vi "Set STG wrapper.vi"(7 "bAckEna":i32, 8 "error in (no error)":errorcluster caption="错误输入（无错误）", 9 "STG_INFO_OBJ In":T1={"uiSenNum"=1, "uiS1TrigerTime"=0, "uiS2TrigerTime"=0, "uiS3TrigerTime"=0} {"uiSenNum" items=["S1"=1, "S2"=2, "S3"=3]}, 10 "dwCanNodeId":u32, 11 "dwDevIndex":u32) -> (0 "error out":errorcluster caption="错误输出", 1 "STG_INFO_OBJ Out":T1={"uiSenNum"=1, "uiS1TrigerTime"=0, "uiS2TrigerTime"=0, "uiS3TrigerTime"=0} {"uiSenNum" items=["S1"=1, "S2"=2, "S3"=3]}, 3 "function return":u32)   [LabVIEW 2016, in "UISimCanFunc_wrapper.lvlib"]
doc: "_declspec (dllexport) DWORD SetSTG_wrapper(DWORD dwDevIndex, DWORD dwCanNodeId,\n P_STG_INFO_OBJ pStgInfoIn, BOOL bAckEna, P_STG_INFO_OBJ pStgInfoOut);"
uses:
  <userlib>/UISimCanFunc_wrapper/UISimCanFunc_wrapper.lvlib
  <userlib>/UISimCanFunc_wrapper/ctl/STG_INFO_OBJ.ctl
  <userlib>/UISimCanFunc_wrapper/UISimCanFunc_wrapper.dll
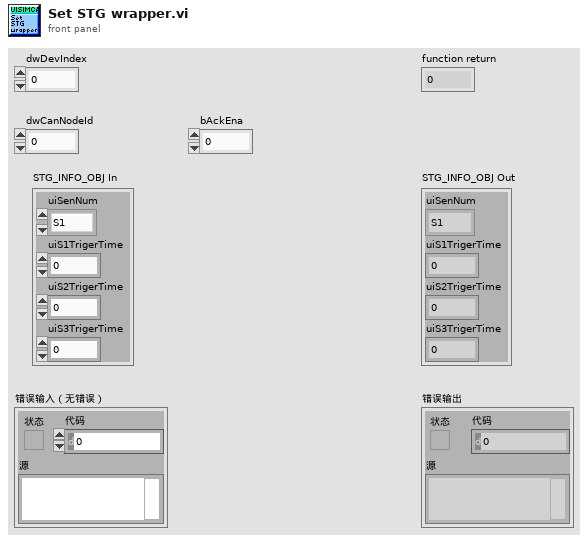
[diagram p1: front panel]
types:
  T1 = typedef "UISimCanFunc_wrapper.lvlib/STG_INFO_OBJ.ctl" = cluster{"uiSenNum":u32, "uiS1TrigerTime":u32, "uiS2TrigerTime":u32, "uiS3TrigerTime":u32}
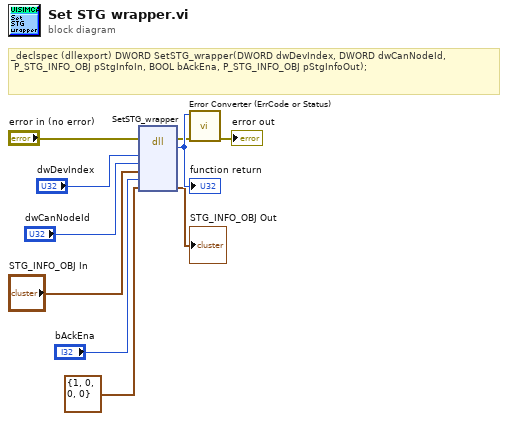
[diagram p0: block diagram]
diagram:
  # "_declspec (dllexport) DWORD SetSTG_wrapper(DWORD dwDevIndex, DWORD dwCanNodeId,\n\tP_STG_INFO_OBJ pStgInfoIn, BOOL bAckEna, P_STG_INFO_OBJ pStgInfoOut);"
  n1 = dll-call lib="C:/Program Files (x86)/National Instruments/LabVIEW 2016/user.lib/UISimCanFunc_wrapper/UISimCanFunc_wrapper.*" fn="SetSTG_wrapper"(error in="error in (no error)", "dwDevIndex"="dwDevIndex", "dwCanNodeId"="dwCanNodeId", "pStgInfoIn"="STG_INFO_OBJ In", "bAckEna"="bAckEna", "pStgInfoOut"=T1 {"uiSenNum"=1, "uiS1TrigerTime"=0, "uiS2TrigerTime"=0, "uiS3TrigerTime"=0} ("STG_INFO_OBJ")) -> (error out=w5:errorcluster, w10:u32, "pStgInfoOut"=→"STG_INFO_OBJ Out":T1)  [unwired: 6 in, 1 out]
  "function return" <- w10
  n2 = call <userlib>:"Error Converter (ErrCode or Status).vi"("error in (no error)"=w5, "error code"=w10) -> ("error out"=→"error out":errorcluster)  [unwired: 9 in]
